vi "publish on demand.vi"(8 "error in":errorcluster, 9 "Data":variant, 10 "Command":string, 11 "node name":string) -> (0 "error out":errorcluster)   [LabVIEW 2020, in "Publisher Subscriber.lvlib"]
uses:
  Publisher Subscriber.lvlib
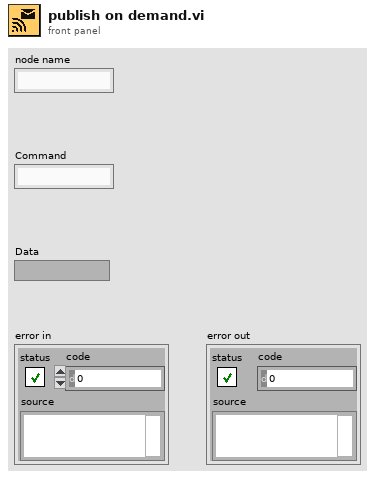
[diagram p1: front panel]
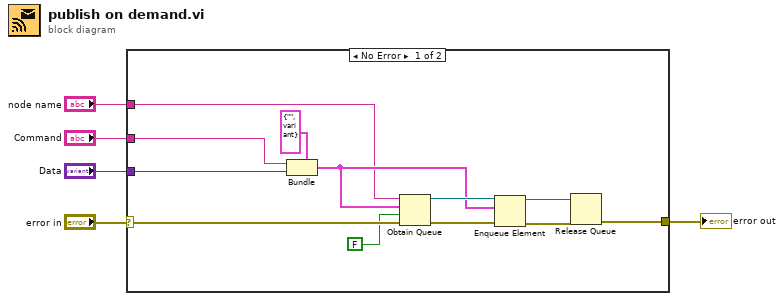
[diagram p0: block diagram]
diagram:
  n1 = case shown="No Error" "error in" {
    selector: "error in" -> [w17 w18]
    tunnel: [w12 w18] -> w4
    tunnel: "Data" -> [w10 _]
    tunnel: "node name" -> [w8 _]
    tunnel: "Command" -> [w7 _]
    frame No Error {
      n2 = Bundle(cluster=cluster{"Command":string, "Data":variant} {"Command"="", "Data"=variant} ("Data Cluster"), "Command"=w7, "Data"=w10) -> (w11:cluster{"Command":string, "Data":variant})
      n3 = Obtain Queue(name (unnamed)=w8, element data type=w11, create if not found? (T)=FALSE, error in (no error)=w17) -> (queue out=w16:refnum<queue>, error out=w15:errorcluster)  [unwired: 1 in, 1 out]
      n4 = Enqueue Element(queue=w16, element=w11, error in (no error)=w15) -> (queue out=w14:refnum<queue>, error out=w13:errorcluster)  [unwired: 1 in, 1 out]
      n5 = Release Queue(queue=w14, error in (no error)=w13) -> (error out=w12:errorcluster)  [unwired: 1 in, 2 out]
    }
    frame Error {
    }
  }
  "error out" <- w4
